vi "test_RemoteDmmSession_CallCloseMeasurementLinkSessionWithDetachBehavior_RemoteSessionDetached.vi"(8 "error in":errorcluster) -> (0 "error out":errorcluster, 2 "result":string, 3 "pass":bool)   [LabVIEW 2020, in "MeasurementServerTests.lvlib"]
uses:
  MeasurementServerTests.lvlib
  Runtime/Sessions/niDMM Sessions/Session Factory/Session Factory.lvclass
  Runtime/Sessions/Instrument Sessions/ISession Factory/Initialize and Close Session Behavior.ctl
  Runtime/Sessions/Instrument Sessions/ISession Factory/ISession Factory.lvclass
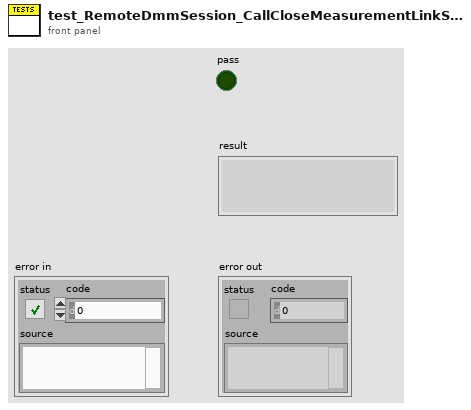
[diagram p1: front panel]
types:
  T1 = typedef "Instrument Sessions.lvlib/ISession Factory.lvclass/Remote Connection Options.ctl" = cluster{"session name":string, "address":string, "port":u32}
  T2 = typedef "Instrument Sessions.lvlib/ISession Factory.lvclass/Initialize and Close Session Behavior.ctl" = enum16{"Initialize and Close", "Attach and Detach", "Initialize and Detach", "Attach and Close"}
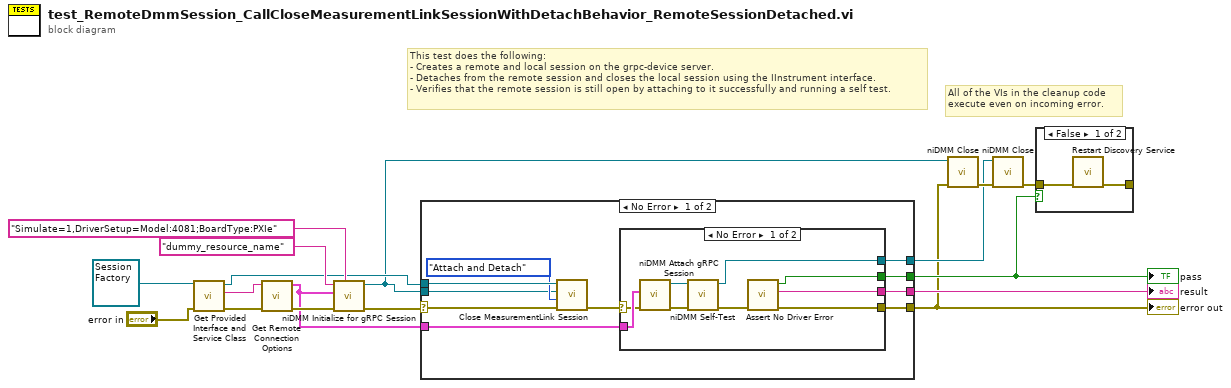
[diagram p0: block diagram]
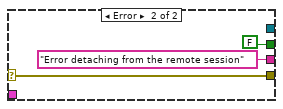
[diagram p2: hidden frame]
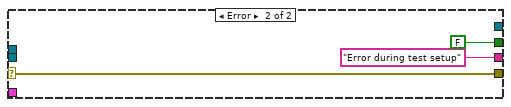
[diagram p3: hidden frame]
diagram:
  # "All of the VIs in the cleanup code\nexecute even on incoming error."
  # "This test does the following:\n- Creates a remote and local session on the grpc-device server.\n- Detaches from the remote session and closes the local session using the IInstrument interface.\n- Verifies that the remote session is still open by attaching to it successfully and running a self test."
  n1 = call-dynamic "Get Provided Interface and Service Class.vi"("error in"="error in", "session factory in"=refnum<class "Session Factory.lvclass"> refnum ("MeasurementLink niDMM.lvlib:Instrument.lvclass")) -> ("error out"=w15:errorcluster, "provided interface"=w14:string, "session factory out"=w10:refnum<class "Session Factory.lvclass">)  [unwired: 6 in, 1 out]
  n2 = call "Get Remote Connection Options.vi"("error in"=w15, "provided interface"=w14) -> ("error out"=w16:errorcluster, "remote connection options"=w9:T1)  [unwired: 8 in]
  n3 = call <instrlib>:"niDMM Initialize for gRPC Session.vi"("Option String"="Simulate=1,DriverSetup=Model:4081;BoardType:PXIe" ("option string"), "error in (no error)"=w16, "gRPC Options"=w9, "Instrument Descriptor"="dummy_resource_name" ("resource name")) -> ("error out"=w11:errorcluster, "instrument handle out"=w4:refnum<k15>)  [unwired: 6 in]
  n4 = case shown="No Error" w11 {
    selector: w11 -> [w27 w41]
    tunnel: w10 -> [w26 _]
    tunnel: w4 -> [w18 _]
    tunnel: w9 -> [w25 _]
    tunnel: [w23 w41] -> w2
    tunnel: [w22 FALSE] -> w5
    tunnel: [w21 "Error during test setup" ("f")] -> w8
    tunnel: [w19 _] -> w3
    frame No Error {
      n5 = call-dynamic "Close MeasurementLink Session.vi"("error in"=w27, "initialize and close session behavior"=Initialize_and_Close_Session_Behavior."Attach and Detach", "session in"=w18, "session factory in"=w26) -> ("error out"=w24:errorcluster)  [unwired: 7 in]
      n6 = case shown="No Error" w24 {
        selector: w24 -> [w35 w37]
        tunnel: w25 -> [w36 _]
        tunnel: [w30 w37] -> w23
        tunnel: [w28 FALSE] -> w22
        tunnel: [w29 "Error detaching from the remote session" ("f")] -> w21
        tunnel: [w32 _] -> w19
        frame No Error {
          n7 = call <instrlib>:"niDMM Attach gRPC Session.vi"("error in (no error)"=w35, "gRPC Options"=w36) -> ("error out"=w33:errorcluster, "instrument handle out"=w34:refnum<k15>)  [unwired: 8 in]
          n8 = call <instrlib>:"niDMM Self-Test.vi"("error in (no error)"=w33, "instrument handle"=w34) -> ("error out"=w31:errorcluster, "instrument handle out"=w32:refnum<k15>)  [unwired: 6 in, 2 out]
          n9 = call "Assert No Driver Error.vi"("error in"=w31) -> ("error out"=w30:errorcluster, "result"=w29:string, "pass?"=w28:bool)  [unwired: 8 in]
        }
        frame Error {
        }
      }
    }
    frame Error {
    }
  }
  "error out" <- w2
  "pass" <- w5
  "result" <- w8
  n10 = call <instrlib>:"niDMM Close.vi"("error in (no error)"=w2, "instrument handle"=w4) -> ("error out"=w7:errorcluster)  [unwired: 9 in]
  n11 = call <instrlib>:"niDMM Close.vi"("error in (no error)"=w7, "instrument handle"=w3) -> ("error out"=w6:errorcluster)  [unwired: 9 in]
  n12 = case shown="False" w5 {
    tunnel: [w44 _] -> _
    tunnel: w6 -> [w43 _]
    frame False {
      n13 = call "Restart Discovery Service.vi"("error in"=w43) -> ("error out"=w44:errorcluster)  [unwired: 10 in]
    }
    frame True {
    }
  }
